vi "Ref Curve Optimize.vi"(7 "linFitOffsetRef":dbl, 8 "error in (no error)":errorcluster caption="错误输入（无错误）", 9 "linFitScalingRef":dbl, 10 "optimize":i32, 11 "asicHandle":i32) -> (0 "error out":errorcluster caption="错误输出", 1 "linFitScalingRef out":dbl, 3 "function return":i32, 5 "linFitOffsetRef out":dbl)   [LabVIEW 2018]
doc: "extern int __stdcall APSxRefCurveOptimize (int asicHandle, IN int optimize, OUT double * linFitScalingRef, OUT double * linFitOffsetRef);"
uses:
  APSx.dll/APSx.dll
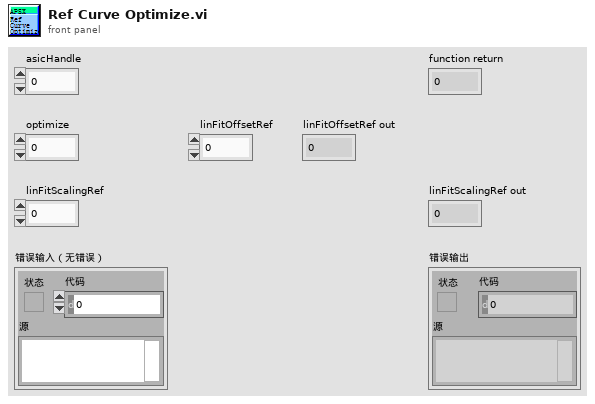
[diagram p1: front panel]
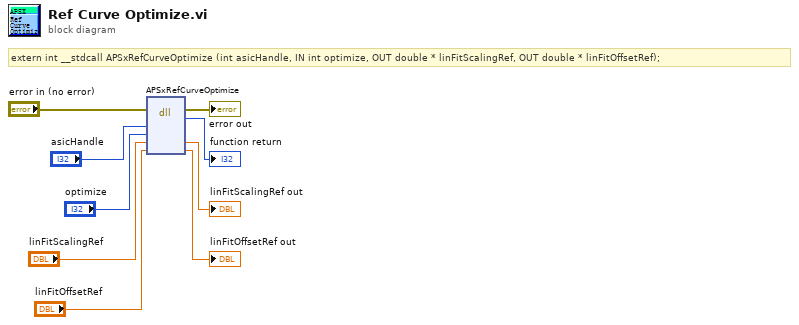
[diagram p0: block diagram]
diagram:
  # "extern int __stdcall APSxRefCurveOptimize (int asicHandle, IN int optimize, OUT double * linFitScalingRef, OUT double * linFitOffsetRef);"
  n1 = dll-call lib="PTH2[abs D项目Feng恒隆项目Labview传感器对中台SourcesAPSx.dllAPSx.*" fn="APSxRefCurveOptimize"(error in="error in (no error)", "asicHandle"="asicHandle", "optimize"="optimize", "linFitScalingRef"="linFitScalingRef", "linFitOffsetRef"="linFitOffsetRef") -> (error out=→"error out":errorcluster, →"function return":i32, "linFitScalingRef"=→"linFitScalingRef out":dbl, "linFitOffsetRef"=→"linFitOffsetRef out":dbl)  [unwired: 4 in, 1 out]
